vi "S2DS_StepCalculation.vi"(0 "Write channel parameters":dbl[](array[numeric]), 1 "Maximum step":i32=600, 2 "Timeout (s)":i32=1000) -> (4 "Step number":u32, 5 "Timed out?":bool, 6 "Values":dbl[](array[numeric]), 7 "Wait time (ms)":u32, 8 "Factor":dbl, 9 "Present value":dbl)   [LabVIEW 2025]
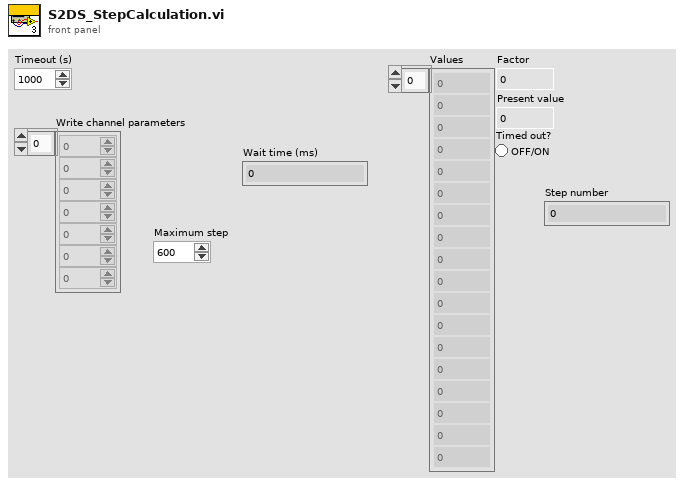
[diagram p1: front panel]
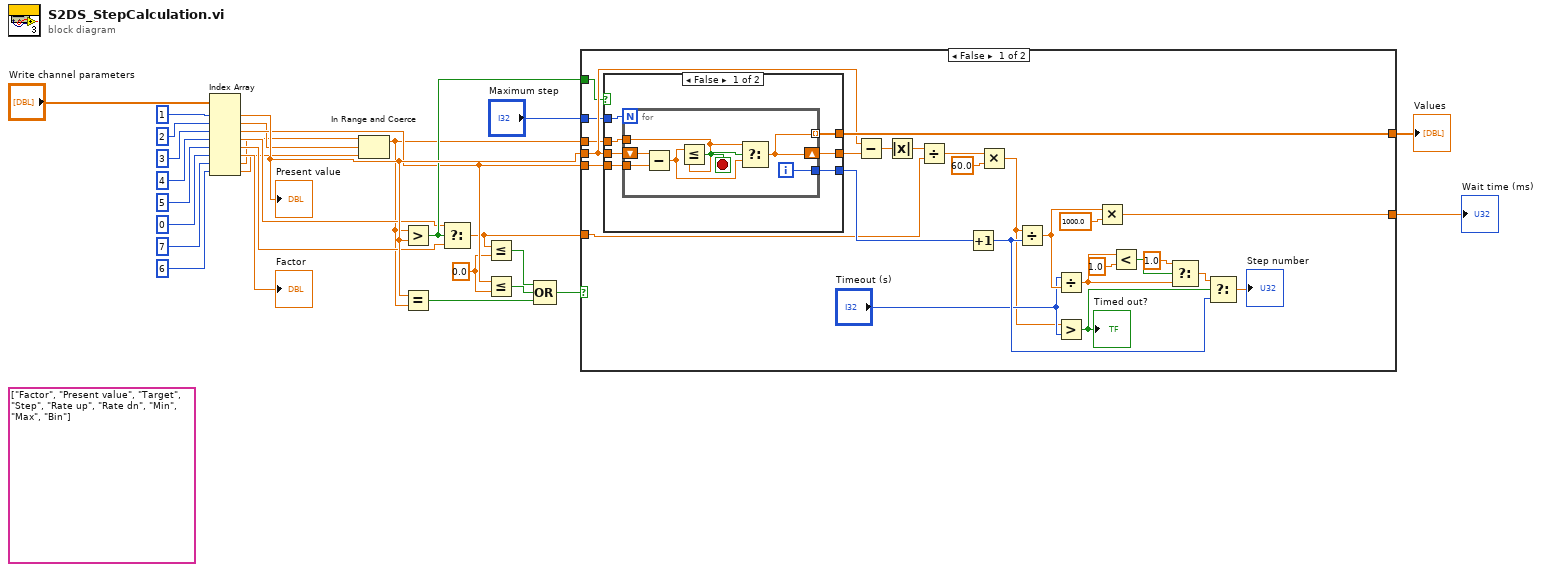
[diagram p0: block diagram]
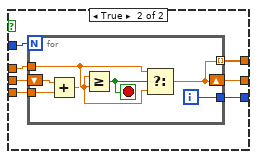
[diagram p2: hidden frame]
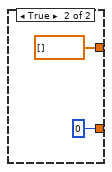
[diagram p3: hidden frame]
diagram:
  (unwired) string[] ["Factor", "Present value", "Target", "Step", "Rate up", "Rate dn", "Min", "Max", "Bin"]
  w13 = 0.0 ("y")
  n1 = Index Array(array="Write channel parameters", index #1=1 ("index"), index #2=2 ("index"), index #3=3 ("index"), index #4=4 ("index"), index #5=5 ("index"), index #6=0 ("index"), index #7=7 ("index"), index #8=6 ("index")) -> (element #1=w18:dbl, element #2=w6:dbl, element #3=w16:dbl, element #4=w15:dbl, element #5=w14:dbl, element #6=→"Factor":dbl, element #7=w3:dbl, element #8=w1:dbl)
  "Present value" <- w18
  n2 = In Range and Coerce(upper limit=w3, x=w6, lower limit=w1) -> (coerced(x)=w5:dbl)  [unwired: 1 out]
  n3 = Greater?(x=w5, y=w18) -> (0:w17:bool)
  n4 = Equal?(x=w18, y=w5) -> (x = y?=w10:bool)
  n5 = Select(t=w15, s=w17, f=w14) -> (s? t:f=w8:dbl)
  n6 = Less Or Equal?(x=w8, y=w13) -> (x <= y?=w12:bool)
  n7 = Less Or Equal?(x=w16, y=w13) -> (x <= y?=w11:bool)
  n8 = Compound Arithmetic op=OR(w12, w11, w10) -> (w9:bool)
  n9 = case shown="False" w9 {
    tunnel: w5 -> [w51 _]
    tunnel: w18 -> [w52 _]
    tunnel: w16 -> [w54 _]
    tunnel: [w53 dbl[] []] -> w25
    tunnel: [w48 0] -> w21
    tunnel: w17 -> [w46 _]
    tunnel: w8 -> [w44 _]
    tunnel: "Maximum step" -> [w43 _]
    frame False {
      n10 = case shown="False" w46 {
        tunnel: w51 -> [w61 w74]
        tunnel: w54 -> [w58 w72]
        tunnel: w52 -> [w59 w73]
        tunnel: [w60 w75] -> w53
        tunnel: [w57 w71] -> w47
        tunnel: w43 -> [w56 w70]
        tunnel: [w55 w69] -> w29
        frame False {
          n11 = for {
            N: w56 -> [_]
            tunnel: [w63] -> w60 mode=indexing
            shift-right: [w63] -> w55
            shift-left: w59 -> [w67]
            tunnel: w58 -> [w68]
            tunnel: w61 -> [w65]
            tunnel: [w62] -> w57
            i -> [w62]
            stop <- w66 stop-if-true
            n12 = Subtract(x=w67, y=w68) -> (x-y=w64:dbl)
            n13 = Less Or Equal?(x=w64, y=w65) -> (x <= y?=w66:bool)
            n14 = Select(t=w65, s=w66, f=w64) -> (s? t:f=w63:dbl)
          }
        }
        frame True {
          n15 = for {
            N: w70 -> [_]
            tunnel: [w77] -> w75 mode=indexing
            shift-right: [w77] -> w69
            shift-left: w73 -> [w81]
            tunnel: w72 -> [w82]
            tunnel: w74 -> [w79]
            tunnel: [w76] -> w71
            i -> [w76]
            stop <- w80 stop-if-true
            n16 = Add(x=w81, y=w82) -> (x+y=w78:dbl)
            n17 = Greater Or Equal?(x=w78, y=w79) -> (x >= y?=w80:bool)
            n18 = Select(t=w79, s=w80, f=w78) -> (s? t:f=w77:dbl)
          }
        }
      }
      n19 = Subtract(x=w52, y=w29) -> (x-y=w50:dbl)
      n20 = Absolute Value(x=w50) -> (abs(x)=w45:dbl)
      n21 = Divide(x=w45, y=w44) -> (x/y=w37:dbl)
      n22 = Increment(x=w47) -> (x+1=w40:i32)
      n23 = Multiply(x=w37, y=60.0) -> (x*y=w35:dbl)
      n24 = Divide(x=w35, y=w40) -> (x/y=w42:dbl)
      n25 = Divide(x="Timeout (s)", y=w42) -> (x/y=w31:dbl)
      n26 = Greater?(x=w35, y="Timeout (s)") -> (0:w41:bool)
      "Timed out?" <- w41
      n27 = Multiply(x=w42, y=1000.0) -> (x*y=w48:dbl)
      n28 = Less?(x=w31, y=1.0) -> (x < y?=w33:bool)
      n29 = Select(t=1.0, s=w33, f=w31) -> (s? t:f=w30:dbl)
      n30 = Select(t=w30, s=w41, f=w40) -> (s? t:f=→"Step number":dbl)
    }
    frame True {
    }
  }
  "Values" <- w25
  "Wait time (ms)" <- w21
